vi "lab1_packet_parser.vi"(10 "preamble bytes":u8[](array[numeric]), 11 "bitstream":i16[](array[numeric])) -> (0 "Found?":bool, 1 "packet counter":u32, 2 "payload length(bytes)":u32, 3 "payload bytes":u8[](array[numeric]))   [LabVIEW 2014]
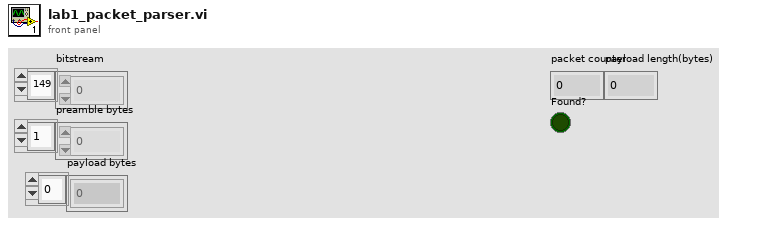
[diagram p1: front panel]
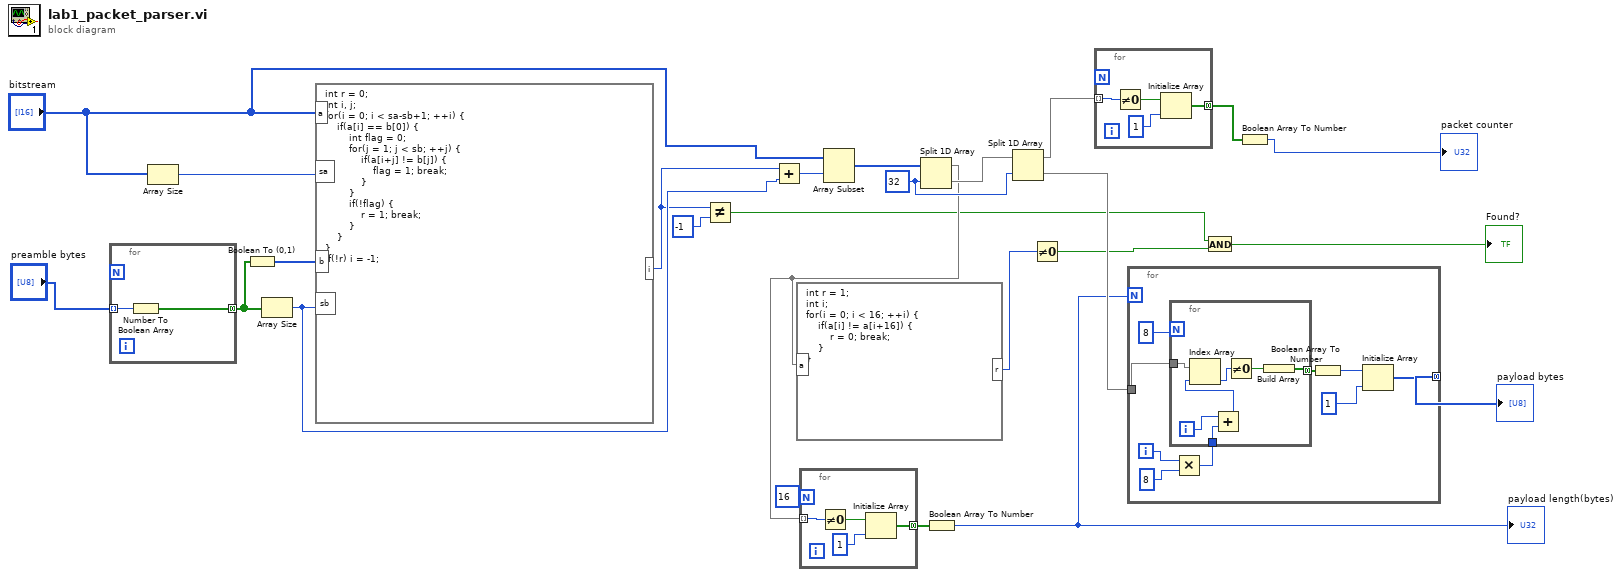
[diagram p0: block diagram]
diagram:
  w16 = 32
  n1 = for {
    tunnel: "preamble bytes" -> [w27] mode=indexing
    tunnel: [w26] -> w24 mode=concatenating
    n2 = Number To Boolean Array(number=w27) -> (Boolean array=w26:bool[])
  }
  n3 = Array Size(array="bitstream") -> (size(s)=w23:i32)
  n4 = Boolean To (0,1)(Boolean=w24) -> (0, 1=w25:i16[])
  n5 = Array Size(array=w24) -> (size(s)=w22:i32)
  n6 = formula code="int r = 0;\nint i, j;\nfor(i = 0; i < sa-sb+1; ++i) {\n    if(a[i] == b[0]) {\n        int flag = 0;\n        for(j = 1; j < sb; ++j) {\n            if(a[i+j] != b[j]) {\n                flag = 1; break;\n            }\n        }\n        if(!flag) {\n            r = 1; break;\n        }\n    }\n}\nif(!r) i = -1;"("b"=w25, "a"="bitstream", "sa"=w23, "sb"=w22) -> ("i"=w21:i32)
  n7 = Not Equal?(x=w21, y=-1) -> (x != y?=w3:bool)
  n8 = Add(x=w21, y=w22) -> (x+y=w7:i32)
  n9 = Array Subset(array="bitstream", index=w7) -> (w19:i16[])  [unwired: 1 in]
  n10 = Split 1D Array(array=w19, index=w16) -> (first subarray=w13:i16[], second subarray=w17:i16[])
  n11 = formula code="int r = 1;\nint i;\nfor(i = 0; i < 16; ++i) {\n    if(a[i] != a[i+16]) {\n        r = 0; break;\n    }\n}"("a"=w13) -> ("r"=w18:i32)
  n12 = for {
    N: 16 -> [_]
    tunnel: w13 -> [w31] mode=indexing
    tunnel: [w29] -> w11 mode=concatenating
    n13 = Not Equal To 0?(x=w31) -> (x != 0?=w30:bool)
    n14 = Initialize Array(w30, 1) -> (w29:bool[])
  }
  n15 = Boolean Array To Number(Boolean array=w11) -> (number=w4:u32)
  "payload length(bytes)" <- w4
  n16 = Split 1D Array(array=w17, index=w16) -> (first subarray=w15:i16[], second subarray=w10:i16[])
  n17 = Not Equal To 0?(x=w18) -> (x != 0?=w2:bool)
  n18 = for {
    tunnel: w15 -> [w35] mode=indexing
    tunnel: [w33] -> w14 mode=concatenating
    n19 = Not Equal To 0?(x=w35) -> (x != 0?=w34:bool)
    n20 = Initialize Array(w34, 1) -> (w33:bool[])
  }
  n21 = for {
    N: w4 -> [_]
    tunnel: w10 -> [w42]
    tunnel: [w40] -> w8 mode=concatenating
    i -> [w38]
    n22 = Multiply(x=w38, y=8) -> (x*y=w36:i32)
    n23 = for {
      N: 8 -> [_]
      tunnel: w42 -> [w46]
      tunnel: [w51] -> w43 mode=concatenating
      tunnel: w36 -> [w48]
      i -> [w49]
      n24 = Add(x=w49, y=w48) -> (x+y=w47:i32)
      n25 = Index Array(array=w46, index=w47) -> (element=w45:i16)
      n26 = Not Equal To 0?(x=w45) -> (x != 0?=w50:bool)
      n27 = Build Array(w50) -> (w51:bool[])
    }
    n28 = Boolean Array To Number(Boolean array=w43) -> (number=w41:u32)
    n29 = Initialize Array(w41, 1) -> (w40:u32[])
  }
  "payload bytes" <- w8
  n30 = And(x=w3, y=w2) -> (x .and. y?=→"Found?":bool)
  n31 = Boolean Array To Number(Boolean array=w14) -> (number=→"packet counter":u32)
